vi "Add VI from File.vi"(8 "error in (no error)":errorcluster, 10 "VI Path":path, 11 "Model in":refnum<class "Model.lvclass">) -> (0 "error out":errorcluster, 3 "Model out":refnum<class "Model.lvclass">)   [LabVIEW 2015, in "Model.lvlib" / "Model.lvclass"]
uses:
  Model.lvclass
  Model Messages/Add VI from Ref Msg/Add VI from Ref Msg.lvclass
  <vilib>/ActorFramework/Actor/Actor.lvclass
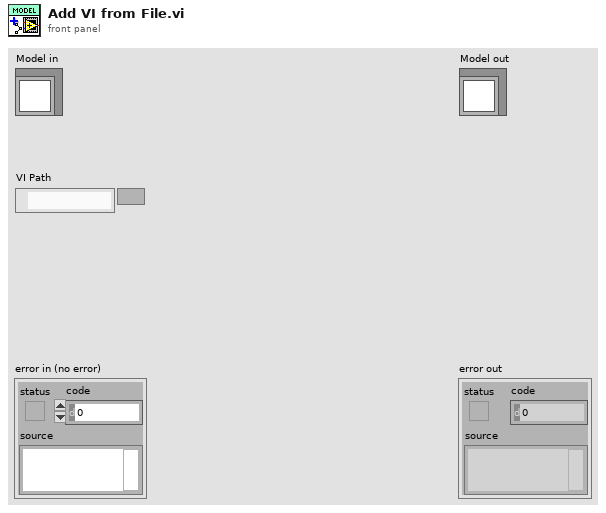
[diagram p1: front panel]
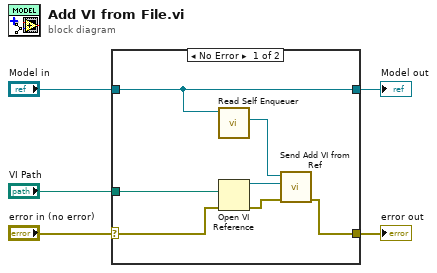
[diagram p0: block diagram]
diagram:
  n1 = case shown="No Error" "error in (no error)" {
    selector: "error in (no error)" -> [w11 w14]
    tunnel: [w6 w14] -> w4
    tunnel: [w8 w13] -> w2
    tunnel: "Model in" -> [w8 w13]
    tunnel: "VI Path" -> [w12 _]
    frame No Error {
      n2 = call <vilib>:"Read Self Enqueuer.vi"("Actor"=w8) -> ("Self Enqueuer"=w7:refnum<class "Message Enqueuer.lvclass">)  [unwired: 10 in]
      n3 = Open VI Reference(vi path=w12, error in (no error)=w11) -> (vi reference=w10:refnum<vi>, error out=w9:errorcluster)  [unwired: 4 in]
      n4 = call "Send Add VI from Ref.vi"("error in (no error)"=w9, "VI Ref"=w10, "Message Enqueuer"=w7) -> ("error out"=w6:errorcluster)  [unwired: 7 in, 1 out]
    }
    frame Error {
    }
  }
  "error out" <- w4
  "Model out" <- w2
